vi "LPA400_parse_response.vi"(0 "Stripped scale response":string="#X01+234") -> (1 "Address":i32, 2 "Weight":dbl format="%.2f", 3 "Error notes":string)   [LabVIEW 2010]
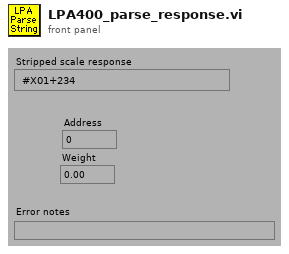
[diagram p1: front panel]
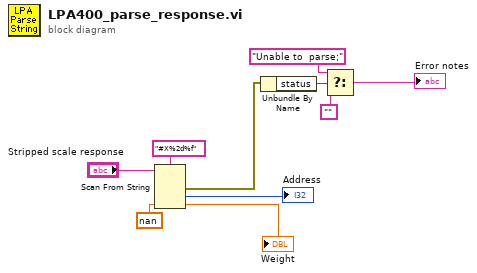
[diagram p0: block diagram]
diagram:
  n1 = Scan From String(format string="#X%2d%f" ("Format String"), input string="Stripped scale response", default 2=nan ("Default Value 2")) -> (error out=w2:errorcluster, output 1=→"Address":i32, output 2=→"Weight":dbl)  [unwired: 2 in, 3 out]
  n2 = Unbundle By Name(w2) -> ("status"=w9:bool)
  n3 = Select(t="Unable to  parse;", s=w9, f="") -> (s? t:f=→"Error notes":string)
